vi "go patten.vi"(11 "controller in":T3) -> (3 "controller out":T3)   [LabVIEW 2016]
uses:
  draw point cluster.ctl
  Classes/Controller/Motion/A3200 Folder/A3200.lvclass
  Classes/Controller/Dispenser/Ultimus V2 Folder/Ultimus V2.lvclass
  Classes/Controller/I-O/NI-DAQ Folder/NI-DAQ.lvclass
  Classes/Controller/Motion/Motion Folder/Motion.lvclass
  Classes/Controller/I-O/I-O Folder/I-O.lvclass
  Classes/Controller/Dispenser/Dispenser Folder/Dispenser.lvclass
panel:
  in  "motion":T1
  in  "dispense":T2={"Vacuum Setting (0000)"=0, "Pressure"=20, "on delay (ms)"=0.5, "off delay (ms) "=0.5} {"Vacuum Setting (0000)" min=0 max=1000 step=1 format="%04.0f"}
  in  "cluster Array input":T4[](array[typedef])
  out "Numeric":dbl=0.237
  out "i":i32=23
  out "size(s)":i32=75
  out "drow point Cluster":T4={"dispense"=FALSE, "Line/circle"=FALSE, "ccw/cw"=FALSE, "pressure"=30.0, "speed"=15.0, "start"=[867.4, 924.5], "end"=[857.4, 924.5], "center"=[6.5, -24.0]}
  in  "use new/data":bool
  in  "file path (dialog if empty)":path=path "D:/Gantry_General/Main/ms_kao/data/CAD PCB full 0.8 P30 20210608/CAD PCB full 0.8 P30 20210608.txt"
  # "使用新/資料"
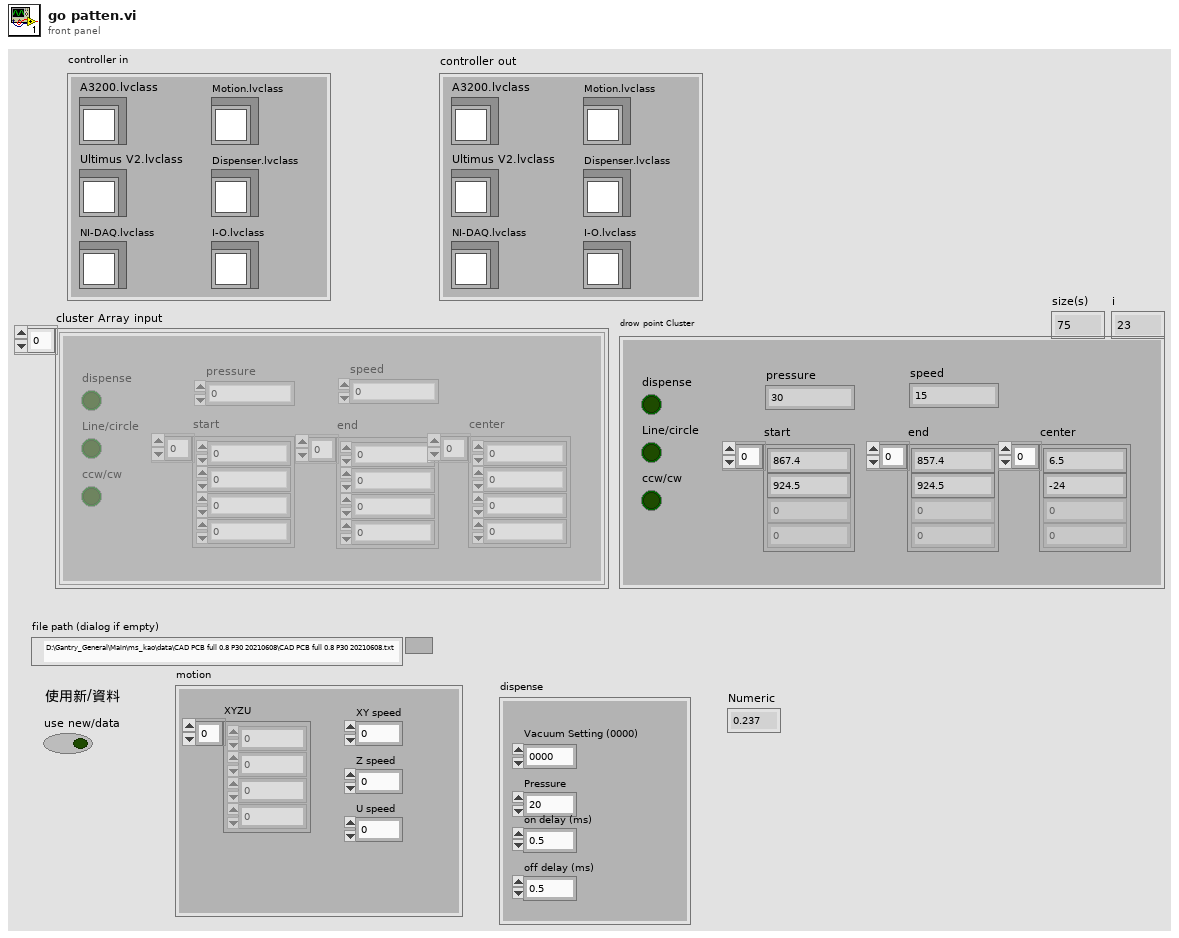
[diagram p1: front panel]
types:
  T1 = cluster{"XYZU ":dbl[], "XY speed":dbl, "Z speed":dbl, "U speed":dbl}
  T2 = cluster{"Vacuum Setting (0000)":i64, "Pressure":i16, "on delay (ms)":dbl, "off delay (ms) ":dbl}
  T3 = cluster{"A3200.lvclass":refnum<class "A3200.lvclass">, "Ultimus V2.lvclass":refnum<class "Ultimus V2.lvclass">, "NI-DAQ.lvclass":refnum<class "NI-DAQ.lvclass">, "Motion.lvclass":refnum<class "Motion.lvclass">, "I-O.lvclass":refnum<class "I-O.lvclass">, "Dispenser.lvclass":refnum<class "Dispenser.lvclass">}
  T4 = typedef "draw point cluster.ctl" = cluster{"dispense":bool, "Line/circle":bool, "ccw/cw":bool, "pressure":dbl, "speed":dbl, "start":dbl[], "end":dbl[], "center":dbl[]}
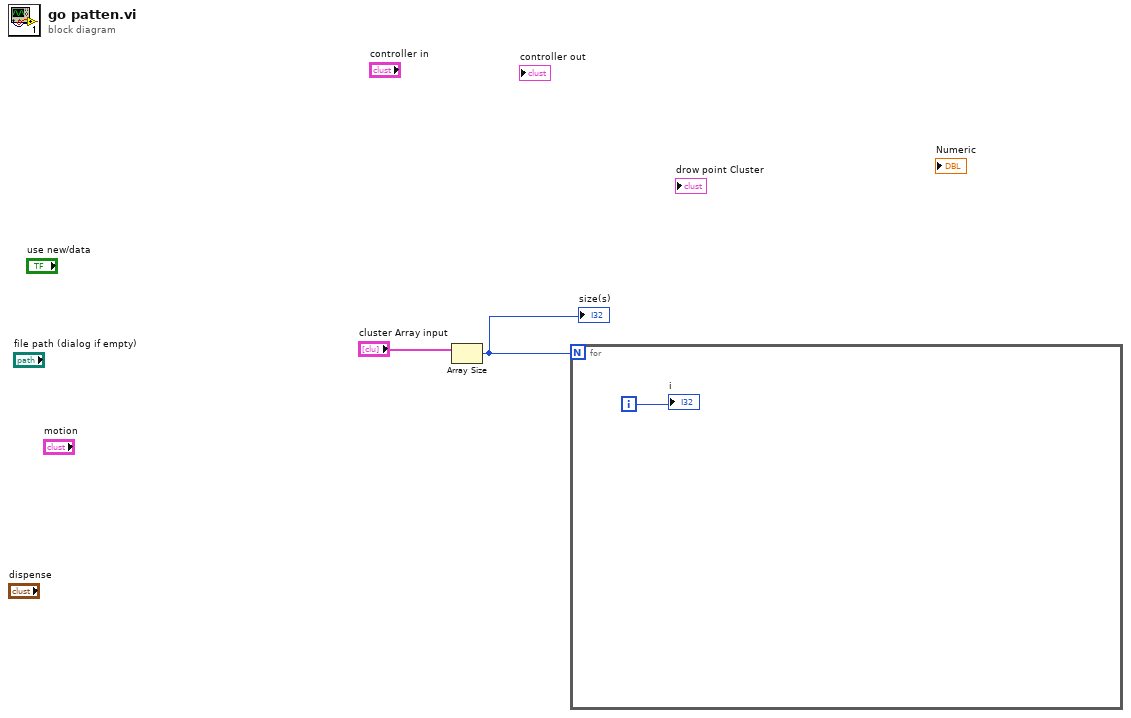
[diagram p0: block diagram]
diagram:
  n1 = Array Size(array="cluster Array input") -> (size(s)=w1:i32)
  "size(s)" <- w1
  n2 = for {
    N: w1 -> [_]
    i -> [w3]
    "i" <- w3
  }
